vi "ConfigureCurrent.vi"(8 "error in (no error)":errorcluster, 10 "Current(0)":dbl, 11 "YP03-60_Y in":refnum<class "YP03-60_Y.lvclass">) -> (0 "error out":errorcluster, 3 "YP03-60_Y out":refnum<class "YP03-60_Y.lvclass">)   [LabVIEW 2020, in "PowerControl.lvlib" / "YP03-60_Y.lvclass"]
uses:
  YP03-60_Y.lvclass
  YP03-60_Y.lvclass/YP03-60_Y.ctl
  <vilib>/Instr/_visa.llb/VISA Configure Serial Port (Instr).vi
  YP03-60_X/YP03-60_X.lvclass
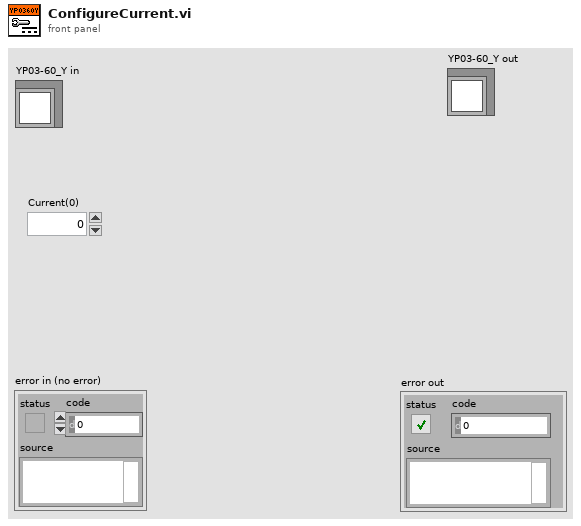
[diagram p1: front panel]
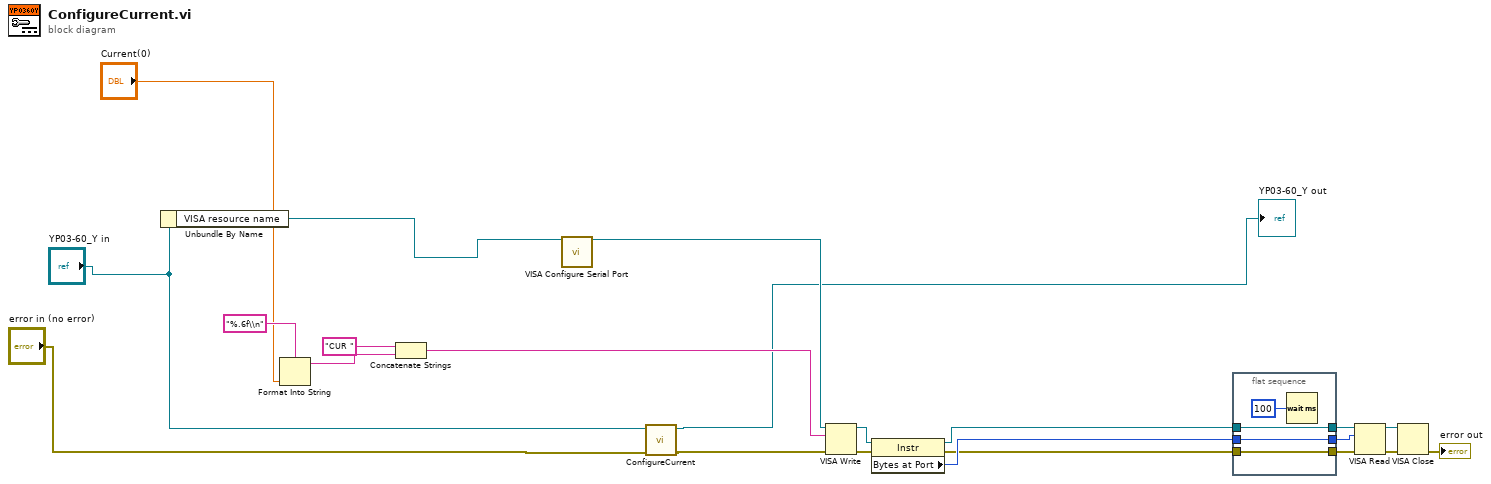
[diagram p0: block diagram]
diagram:
  n1 = Unbundle By Name("YP03-60_Y in") -> ("VISA resource name"=w1:refnum<visa-resource-name>)
  n2 = Format Into String(format string="%.6f\\n", "Current(0)") -> (resulting string=w13:string)  [unwired: 2 in, 1 out]
  n3 = Concatenate Strings("CUR " ("string"), w13) -> (w16:string)
  n4 = call-poly "VISA Configure Serial Port"("VISA resource name"=w1) -> ("VISA resource name out"=w19:refnum<visa-resource-name>)  [unwired: 13 in, 1 out]
  n5 = call-parent "ConfigureCurrent.vi"("error in (no error)"="error in (no error)", "YP03-60_X in"="YP03-60_Y in") -> ("error out 2"=w5:errorcluster, "YP03-60_X out"=→"YP03-60_Y out":refnum<class "YP03-60_Y.lvclass">)  [unwired: 8 in]
  n6 = VISA Write(VISA resource name=w19, write buffer=w16, error in (no error)=w5) -> (VISA resource name out=w17:refnum<visa-resource-name>, error out=w18:errorcluster)  [unwired: 1 out]
  n7 = property class="Instr"(reference=w17, error in=w18) -> (reference out=w10:refnum<visa-resource-name>, error out=w8:errorcluster, "Bytes at Port"=w12:u32)
  n8 = flat-sequence {
    tunnel: w10 -> [w26]
    tunnel: [w26] -> w9
    tunnel: [w25] -> w7
    tunnel: w8 -> [w25]
    tunnel: [w24] -> w11
    tunnel: w12 -> [w24]
    frame #0 {
      n9 = Wait (ms)(milliseconds to wait=u32 100) -> ()  [unwired: 1 out]
    }
  }
  n10 = VISA Read(VISA resource name=w9, byte count=w11, error in (no error)=w7) -> (VISA resource name out=w20:refnum<visa-resource-name>, error out=w22:errorcluster)  [unwired: 2 out]
  n11 = VISA Close(VISA resource name=w20, error in (no error)=w22) -> (error out=→"error out":errorcluster)
